vi "Create Queue.vi"(8 "error in (no error)":errorcluster, 9 "Region":T1, 10 "Name":string, 11 "AWS Credentials":T2) -> (0 "error out":errorcluster, 3 "SQS":refnum<class "SQS.lvclass">)   [LabVIEW 2015, in "NI_SQS.lvlib" / "SQS.lvclass"]
uses:
  SQS.lvclass
  Core/AWS Credentials.ctl
  Core/Region.ctl
  Core/Request Options.ctl
  Core/Name Value Pair.ctl
  Core/AWS Core_class/AWS Core.lvclass/AWS Core.ctl
  SQS.lvclass/SQS.ctl
  Core/AWS Core_class/Write Credentials.vi
  Core/AWS Core_class/Write Region.vi
  Core/AWS Core_class/Write Service.vi
  Core/AWS Core_class/Write Verify Server.vi
  Write Account Number.vi
  Write Name.vi
  Write URL.vi
  Core/NI_AWS Core.lvlib
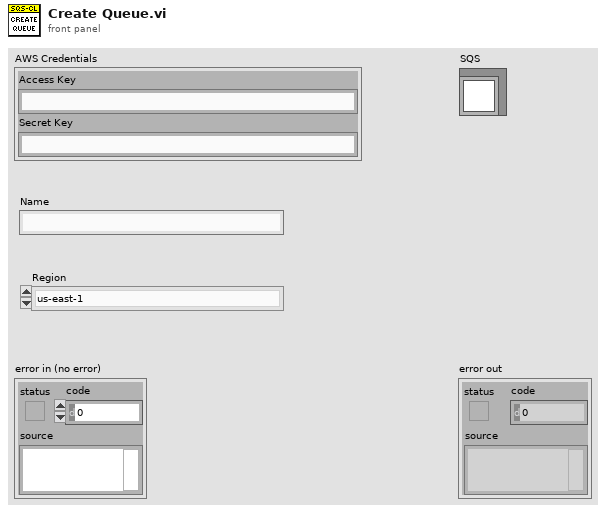
[diagram p1: front panel]
types:
  T1 = typedef "NI_AWS Core.lvlib/Region.ctl" = enum16{"us-east-1", "us-east-2", "us-west-1", "us-west-2", "ap-northeast-1", "ap-northeast-2", "ap-southeast-1", "ap-southeast-2", "ca-central-1", "eu-central-1", "eu-west-1", "eu-west-2", "sa-east-1"}
  T2 = typedef "NI_AWS Core.lvlib/AWS Credentials.ctl" = cluster{"Access Key":string, "Secret Key":string}
  T3 = typedef "NI_AWS Core.lvlib/Name Value Pair.ctl" = cluster{"name":string, "value":string}
  T4 = typedef "NI_AWS Core.lvlib/Request Options.ctl" = cluster{"request headers":T3[], "request parameters":T3[], "request body":string}
  T5 = typedef "NI_AWS Core.lvlib/Response.ctl" = cluster{"Headers":string, "Body":string}
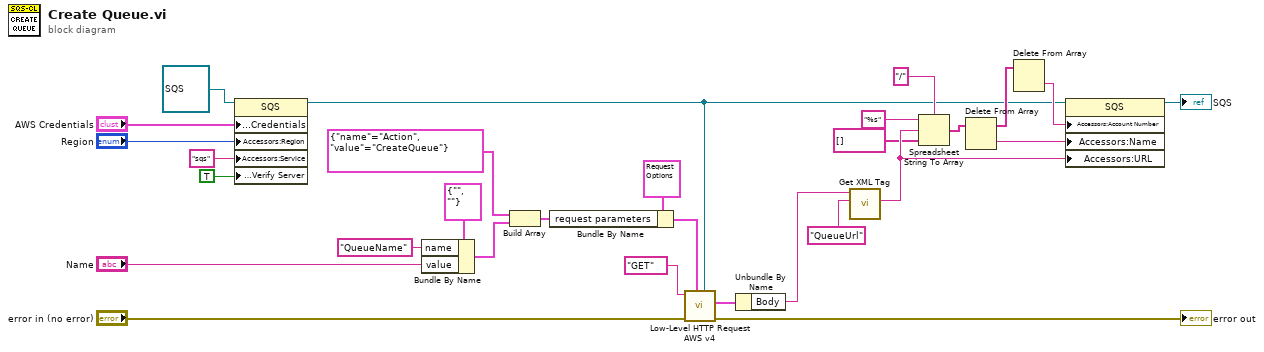
[diagram p0: block diagram]
diagram:
  n1 = property class="SQS"(reference=refnum<class "SQS.lvclass"> refnum ("NI_SQS.lvlib:SQS"), "Accessors:Credentials"="AWS Credentials", "Accessors:Region"="Region", "Accessors:Service"="sqs" ("Service"), "Accessors:Verify Server"=TRUE ("Verify Server")) -> (reference out=w8:refnum<class "SQS.lvclass">)  [unwired: 1 in, 1 out]
  n2 = Bundle By Name(cluster=T3 {"name"="", "value"=""} ("element"), "name"="QueueName", "value"="Name") -> (w1:T3)
  n3 = Build Array(T3 {"name"="Action", "value"="CreateQueue"} ("Name Value Pair"), w1) -> (w6:T3[])
  n4 = Bundle By Name(cluster=T4 {"request headers"=[], "request parameters"=[{"name"="Action", "value"="ListQueues"}], "request body"=""} ("Request Options"), "request parameters"=w6) -> (w24:T4)
  n5 = call "Low-Level HTTP Request AWS v4.vi"("AWS Core"=w8, "Request Options"=w24, "error in (no error)"="error in (no error)", "HTTP-Verb"="GET") -> ("error out"=→"error out":errorcluster, "Response"=w10:T5)  [unwired: 5 in, 1 out]
  n6 = Unbundle By Name(w10) -> ("Body"=w9:string)
  n7 = call "Get XML Tag.vi"("Tag name"="QueueUrl", "XML String in"=w9) -> ("Tag value"=w18:string)  [unwired: 5 in, 4 out]
  n8 = Spreadsheet String To Array(delimiter (Tab)="/", format string="%s", spreadsheet string=w18, array type (2D Dbl)=string[] []) -> (array=w14:string[])
  n9 = Delete From Array(array=w14) -> (deleted portion=w13:string, array with subset deleted=w12:string[])  [unwired: 2 in]
  n10 = Delete From Array(array=w12) -> (deleted portion=w11:string)  [unwired: 2 in, 1 out]
  n11 = property class="SQS"(reference=w8, "Accessors:Account Number"=w11, "Accessors:Name"=w13, "Accessors:URL"=w18) -> (reference out=→"SQS":refnum<class "SQS.lvclass">)  [unwired: 1 in, 1 out]
